vi "Build Filter.vi"(8 "error in (no error)":errorcluster, 11 "Filter Config Display in":refnum<class "Filter Config Display.lvclass">) -> (0 "error out":errorcluster, 3 "Filter Config Display out":refnum<class "Filter Config Display.lvclass">)   [LabVIEW 2016, in "Assert API Components.lvlib" / "Assert Display.lvlib" / "Filter Config Display.lvlib" / "Filter Config Display.lvclass"]
uses:
  Filter Config Display.lvclass
  C:/Program Files (x86)/National Instruments/LabVIEW 2016/vi.lib/ActorFramework/Actor/Actor.lvclass
  Assert Display/Assert Display/Item Configuration.ctl
  Service Config Display/Service Config Display/Items.ctl
  <vilib>/ActorFramework/Actor/Actor.lvclass/Actor.ctl
  Filter Config Display.lvclass/Filter Config Display.ctl
  Assert Display/Assert Display Messages/New Item Msg/New Item Msg.lvclass/New Item Msg.ctl
  <vilib>/ActorFramework/Message Enqueuer/Message Enqueuer.lvclass/Message Enqueuer.ctl
  <vilib>/ActorFramework/Message Enqueuer/Enqueue.vi
  Assert Display/Assert Display Messages/New Item Msg/New Item Msg.lvclass
  C:/Program Files (x86)/National Instruments/LabVIEW 2016/vi.lib/ActorFramework/Message/Message.lvclass
  <vilib>/Utility/LVClass/Get LV Class Name.vi
  <resource>/AFDebug/Generate Trace for Message.vi
  <vilib>/ActorFramework/Message Priority Queue/Priority Enqueue.vi
  <vilib>/ActorFramework/Actor/Actor.lvclass
  Assert Display/Assert Display.lvlib
  Assert API Components/Filter Configurations/Base Filter.lvclass
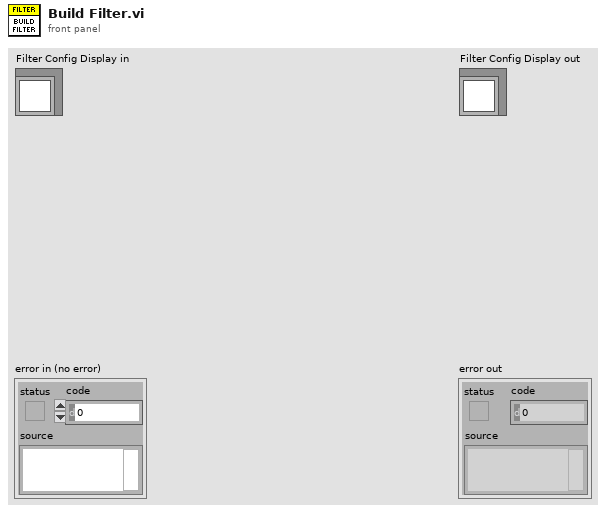
[diagram p1: front panel]
types:
  T1 = typedef "Assert API Components.lvlib/Assert Display.lvlib/Item Configuration.ctl" = cluster{"Item Type":T2, "Configuration":variant}
  T2 = typedef "Assert API Components.lvlib/Assert Display.lvlib/Items.ctl" = enum16{"Service", "Filter"}
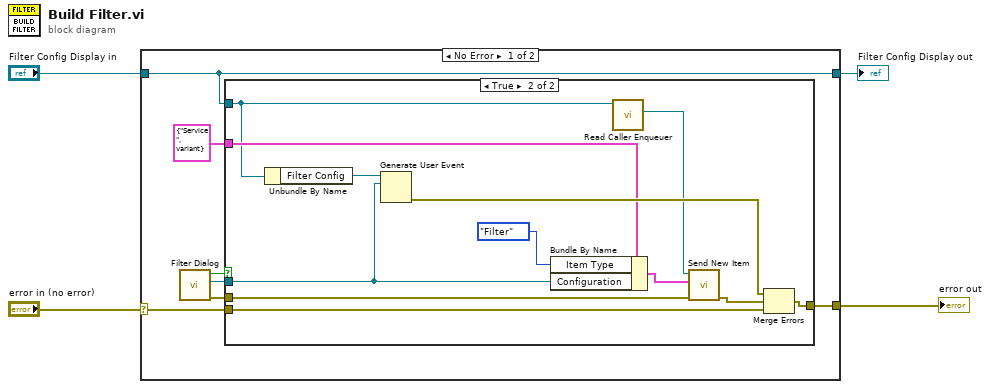
[diagram p0: block diagram]
diagram:
  n1 = case shown="No Error" "error in (no error)" {
    selector: "error in (no error)" -> [w11 w26]
    tunnel: [w6 w26] -> w3
    tunnel: [w10 w25] -> w1
    tunnel: "Filter Config Display in" -> [w10 w25]
    frame No Error {
      n2 = call "Filter Dialog.vi"() -> ("error out"=w7:errorcluster, "Base Filter out"=w8:refnum<class "Base Filter.lvclass">, "Valid Filter Configuration"=w5:bool)  [unwired: 9 in]
      n3 = case shown="True" w5 {
        tunnel: w11 -> [w12 w23]
        tunnel: w10 -> [_ w15]
        tunnel: T1 {"Item Type"=enum."Service", "Configuration"=variant} ("Item Configuration") -> [_ w22]
        tunnel: w8 -> [_ w13]
        tunnel: w7 -> [_ w20]
        tunnel: [w12 w19] -> w6
        frame False {
        }
        frame True {
          n4 = Unbundle By Name(w15) -> ("Filter Config"=w14:refnum<user-event>)
          n5 = Generate User Event(user event=w14, event data cluster=w13) -> (error out=w24:errorcluster)  [unwired: 2 in, 1 out]
          n6 = Bundle By Name(cluster=w22, "Item Type"=Items."Filter", "Configuration"=w13) -> (w21:T1)
          n7 = call <vilib>:"Read Caller Enqueuer.vi"("Actor"=w15) -> ("Caller Enqueuer"=w17:refnum<class "Message Enqueuer.lvclass">)  [unwired: 10 in]
          n8 = call "Send New Item.vi"("error in (no error)"=w20, "Item Configuration"=w21, "Message Enqueuer"=w17) -> ("error out"=w18:errorcluster)  [unwired: 7 in, 1 out]
          n9 = Merge Errors(w24, w18, w23) -> (w19:errorcluster)
        }
      }
    }
    frame Error {
    }
  }
  "error out" <- w3
  "Filter Config Display out" <- w1
